vi "Disabled Sites Offset Dialog.vi"(8 "error in":errorcluster, 10 "Disabled Sites":i32[](array[numeric])) -> (0 "error out":errorcluster, 2 "Offset Update Option Out":enum32{"Use Original Offset", "Use New Offset"}(ring), 3 "New Offset  Out":dbl)   [LabVIEW 2020, in "GUCalibration2.lvlib"]
uses:
  GUCalibration2.lvlib
  Controls/User Facing Msg Enum.ctl
panel:
  out "String":string
  in  "Offset Update Option":enum32{"Use Original Offset", "Use New Offset"}(radio)
  in  "OK":bool
  in  "New Offset":dbl
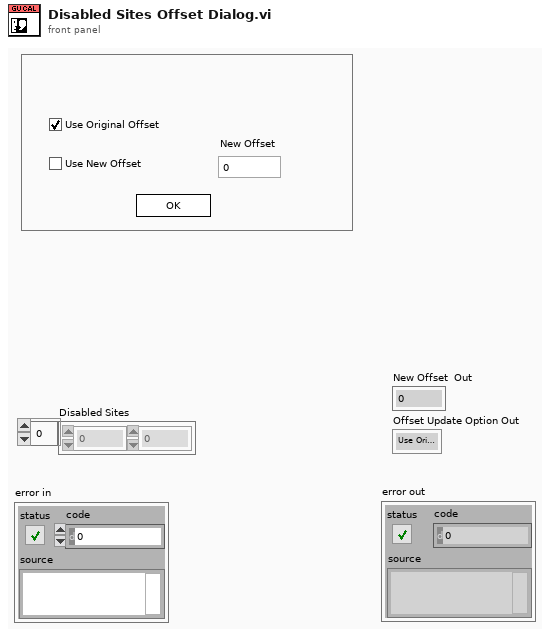
[diagram p1: front panel]
types:
  T1 = typedef "GUCalibration2.lvlib/User Facing Msg Enum.ctl" = enum16{"Invalid GU Number", "Select More GU", "Exceptional Lot End", "Not All Sites Test", "GU Arrange Error", "Put GU In Sites", "No Cal Site Offset Msg"}
  T2 = enum8{"Enabled", "Disabled", "Disabled and Grayed Out"}
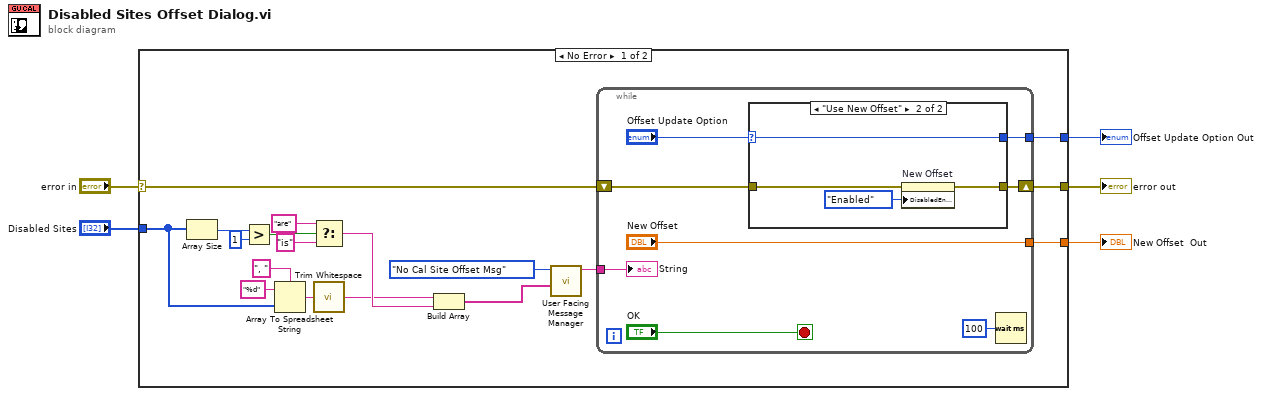
[diagram p0: block diagram]
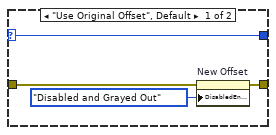
[diagram p2: hidden frame]
diagram:
  n1 = case shown="No Error" "error in" {
    selector: "error in" -> [w9 w40]
    tunnel: [w8 w40] -> w4
    tunnel: "Disabled Sites" -> [w23 _]
    tunnel: [w7 _] -> w2
    tunnel: [w6 _] -> w1
    frame No Error {
      n2 = Array Size(array=w23) -> (size(s)=w22:i32)
      n3 = Greater?(x=w22, y=1) -> (0:w20:bool)
      n4 = Array To Spreadsheet String(delimiter (Tab)=", ", array=w23, 3:"%d" ("format string")) -> (spreadsheet string=w15:string)
      n5 = Select(t="are", s=w20, f="is") -> (s? t:f=w12:string)
      n6 = call <vilib>:"Trim Whitespace.vi"("string"=w15) -> ("trimmed string"=w11:string)  [unwired: 1 in]
      n7 = Build Array(w11, w12) -> (w13:string[])
      n8 = call "User Facing Message Manager.vi"("Variable Msg"=w13, "User Facing Msg"=User_Facing_Msg_Enum."No Cal Site Offset Msg") -> ("User Facing Msg Out"=w10:string)  [unwired: 7 in, 2 out]
      n9 = while {
        tunnel: ["New Offset"] -> w7
        tunnel: [w24] -> w6
        tunnel: w10 -> [w28]
        shift-right: [w26] -> w8
        shift-left: w9 -> [w27]
        stop <- "OK" stop-if-true
        n10 = case shown="\"Use New Offset\"" "Offset Update Option" {
          selector: "Offset Update Option" -> [w32 w36]
          tunnel: w27 -> [w35 w39]
          tunnel: [w34 w38] -> w26
          tunnel: [w32 w36] -> w24
          frame "Use Original Offset", Default {
            n11 = property on="New Offset" class="DigNum (strict)"(error in=w35, "DisabledEnum"=T2."Disabled and Grayed Out" ("Disabled")) -> (error out=w34:errorcluster)  [unwired: 1 in, 1 out]
          }
          frame "Use New Offset" {
            n12 = property on="New Offset" class="DigNum (strict)"(error in=w39, "DisabledEnum"=T2."Enabled" ("Disabled")) -> (error out=w38:errorcluster)  [unwired: 1 in, 1 out]
          }
        }
        n13 = Wait (ms)(milliseconds to wait=u32 100) -> ()  [unwired: 1 out]
        "String" <- w28
      }
    }
    frame Error {
    }
  }
  "error out" <- w4
  "New Offset  Out" <- w2
  "Offset Update Option Out" <- w1
